vi "HIOKI PW3390 Conf Measure Item Harmonic.vi"(0 "VISA Resource":refnum<visa-resource-name>, 1 "LIST":T1={"LIST1"=[FALSE, FALSE, FALSE, FALSE, FALSE, FALSE, FALSE, FALSE], "LIST2"=[FALSE, FALSE, FALSE, FALSE, FALSE, FALSE, FALSE, FALSE], "LIST1 2"=[FALSE, FALSE, FALSE, FALSE, FALSE, FALSE, FALSE, FALSE], "LIST2 2"=[FALSE, FALSE, FALSE, FALSE, FALSE, FALSE, FALSE], "LIST1 3"=[FALSE, FALSE, FALSE, FALSE, FALSE, FALSE, FALSE, FALSE], "LIST2 3"=[FALSE, FALSE, FALSE, FALSE, FALSE, FALSE, FALSE]}, 2 "Min Order (0)":i32 min=0 max=100, 3 "Max Order (100)":i32=100 min=0 max=100, 4 "ODD/EVEN/ALL (2: ALL)":enum16{"ODD", "EVEN", "ALL"}(ring)=enum."ALL", 5 "error in (no error)":errorcluster, 6 "Set/Query (F: Set)":bool, 7 "OPC query (T: ON)":bool=TRUE, 8 "All Clear (F: Off)":bool, 9 "Error Out (F: Off)":bool) -> (14 "VISA Resource out":refnum<visa-resource-name>, 15 "LIST out":T1, 16 "Min Order out":i32, 17 "Max Order out":i32=100, 18 "ODD/EVEN/ALL out":enum16{"ODD", "EVEN", "ALL"}(ring)=enum."ALL", 19 "error out":errorcluster)   [LabVIEW 2009]
doc: "Set/Query\n Set: Send the setting commands for the device.\n Query: Query the setting of the device.\n\nAll Clear\n Initializes the harmonic communication output data items.\n All harmonic communication output data items become OFF.\n\nList\n Specify the Harmonic List (Level, Content, Phase Angle) .\n\nMin Order\n Sets the lower order value.\n Input Range: 0 - 100\nMax Order\n Sets the upper order value.\n Input Range: 0 - 100\n\nODD/EVEN/ALL\n Sets the harmonic order to output."
panel:
  # "Order"
  # "Order out"
  # "U1"
  # "U2"
  # "U3"
  # "U4"
  # "I1"
  # "I2"
  # "I3"
  # "I4"
  # "Level"
  # "P12"
  # "P123"
  # "P1"
  # "P2"
  # "P3"
  # "P4"
  # "P34"
  # "FREQ"
  # "U1"
  # "U2"
  # "U3"
  # "U4"
  # "I1"
  # "I2"
  # "I3"
  # "I4"
  # "%"
  # "P12"
  # "P123"
  # "P1"
  # "P2"
  # "P3"
  # "P4"
  # "P34"
  # "U1"
  # "U2"
  # "U3"
  # "U4"
  # "I1"
  # "I2"
  # "I3"
  # "I4"
  # "Phase"
  # "P12"
  # "P123"
  # "P1"
  # "P2"
  # "P3"
  # "P4"
  # "P34"
  # "U1"
  # "U2"
  # "U3"
  # "U4"
  # "I1"
  # "I2"
  # "I3"
  # "I4"
  # "Level"
  # "P12"
  # "P123"
  # "P1"
  # "P2"
  # "P3"
  # "P4"
  # "P34"
  # "FREQ"
  # "U1"
  # "U2"
  # "U3"
  # "U4"
  # "I1"
  # "I2"
  # "I3"
  # "I4"
  # "%"
  # "P12"
  # "P123"
  # "P1"
  # "P2"
  # "P3"
  # "P4"
  # "P34"
  # "U1"
  # "U2"
  # "U3"
  # "U4"
  # "I1"
  # "I2"
  # "I3"
  # "I4"
  # "Phase"
  # "P12"
  # "P123"
  # "P1"
  # "P2"
  # "P3"
  # "P4"
  # "P34"
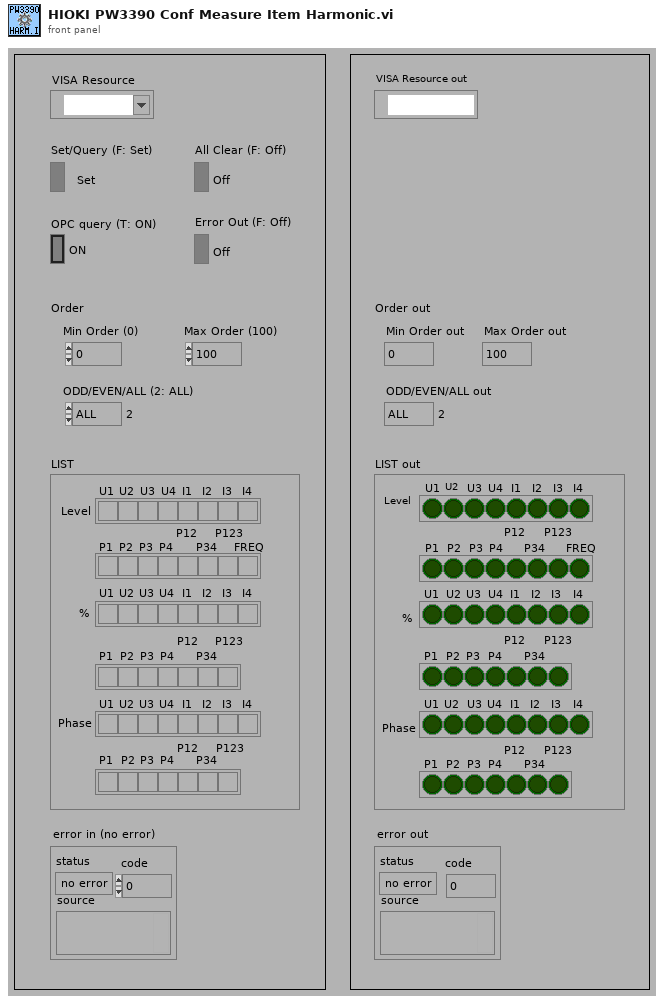
[diagram p1: front panel]
types:
  T1 = cluster{"LIST1":bool[], "LIST2":bool[], "LIST1 2":bool[], "LIST2 2":bool[], "LIST1 3":bool[], "LIST2 3":bool[]}
  T2 = cluster{"Boolean array":bool[], "Boolean array":bool[], "Boolean array":bool[], "Boolean array":bool[], "Boolean array":bool[], "Boolean array":bool[]}
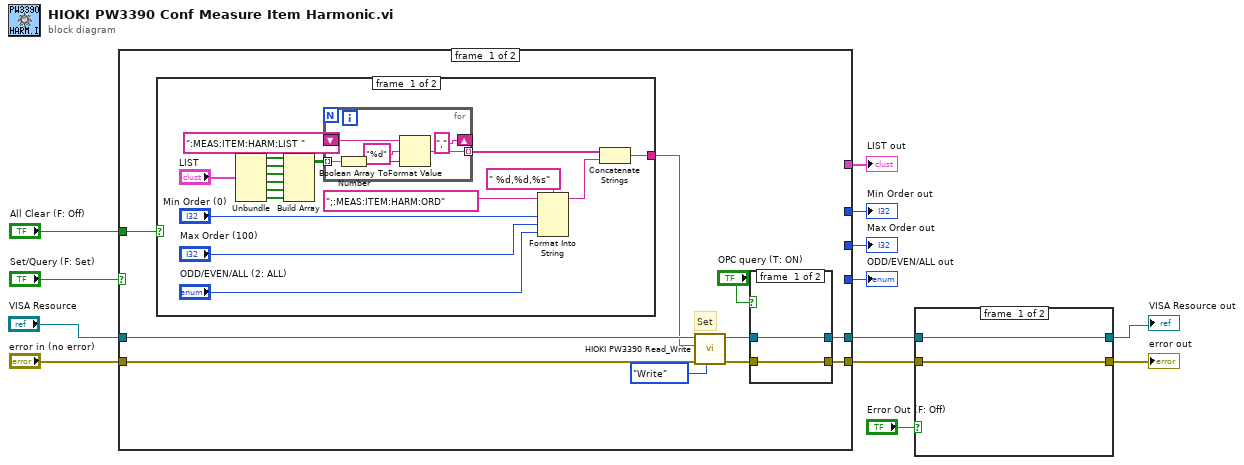
[diagram p0: block diagram]
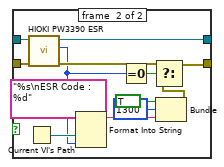
[diagram p2: hidden frame]
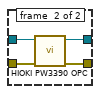
[diagram p3: hidden frame]
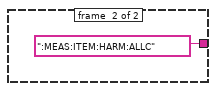
[diagram p4: hidden frame]
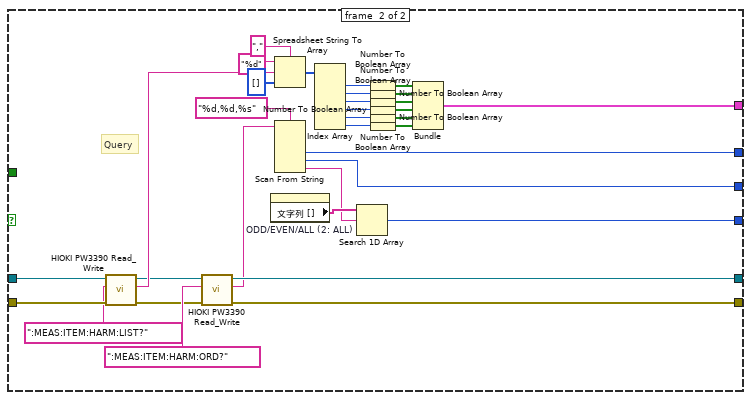
[diagram p5: hidden frame]
diagram:
  n1 = case shown="FALSE" "Set/Query (F: Set)" {
    tunnel: "error in (no error)" -> [w22 w85]
    tunnel: [w14 w78] -> w10
    tunnel: "VISA Resource" -> [w23 w86]
    tunnel: [w15 w75] -> w9
    tunnel: [_ w61] -> w7
    tunnel: [_ w56] -> w6
    tunnel: [_ w55] -> w5
    tunnel: [_ w54] -> w4
    tunnel: "All Clear (F: Off)" -> [w19 _]
    frame #0 {
      # "Set"
      n2 = case shown="FALSE" w19 {
        tunnel: [w30 ":MEAS:ITEM:HARM:ALLC"] -> w20
        frame #0 {
          n3 = Unbundle("LIST") -> ("LIST1"=w43:bool[], "LIST2"=w42:bool[], "LIST1 2"=w41:bool[], "LIST2 2"=w40:bool[], "LIST1 3"=w39:bool[], "LIST2 3"=w38:bool[])
          n4 = Build Array(w43, w42, w41, w40, w39, w38) -> (w46:bool[][])
          n5 = for {
            shift-right: [","] -> _
            shift-left: ":MEAS:ITEM:HARM:LIST " -> [w47]
            tunnel: [w48] -> w35 mode=indexing
            tunnel: w46 -> [w51] mode=indexing
            n6 = Boolean Array To Number(Boolean array=w51) -> (number=w50:u32)
            n7 = Format Value(string ("")=w47, format string="%d", value (0)=w50) -> (output string=w48:string)
          }
          n8 = Format Into String(format string=" %d,%d,%s", initial string=";:MEAS:ITEM:HARM:ORD", "Min Order (0)", "Max Order (100)", "ODD/EVEN/ALL (2: ALL)") -> (resulting string=w31:string)  [unwired: 1 in, 1 out]
          n9 = Concatenate Strings(w35, w31) -> (w30:string)
        }
        frame #1 {
        }
      }
      n10 = call <instrlib>:"HIOKI PW3390 Read_Write.vi"("Read/Write"=enum16{"Read", "Write"}."Write", "error in (no error)"=w22, "data in"=w20, "VISA Resource"=w23) -> ("error out"=w16:errorcluster, "VISA Resource out"=w17:refnum<visa-resource-name>)  [unwired: 5 in, 1 out]
      n11 = case shown="TRUE" "OPC query (T: ON)" {
        tunnel: [w25 w29] -> w15
        tunnel: [w24 w28] -> w14
        tunnel: w17 -> [w25 w27]
        tunnel: w16 -> [w24 w26]
        frame #0 {
        }
        frame #1 {
          n12 = call <instrlib>:"HIOKI PW3390 OPC.vi"("error in (no error)"=w26, "VISA Resource"=w27) -> ("error out"=w28:errorcluster, "VISA Resource out"=w29:refnum<visa-resource-name>)  [unwired: 7 in, 1 out]
        }
      }
    }
    frame #1 {
      # "Query"
      n13 = call <instrlib>:"HIOKI PW3390 Read_Write.vi"("error in (no error)"=w85, "data in"=":MEAS:ITEM:HARM:LIST?", "VISA Resource"=w86) -> ("error out"=w76:errorcluster, "data out"=w82:string, "VISA Resource out"=w77:refnum<visa-resource-name>)  [unwired: 6 in]
      n14 = call <instrlib>:"HIOKI PW3390 Read_Write.vi"("error in (no error)"=w76, "data in"=":MEAS:ITEM:HARM:ORD?", "VISA Resource"=w77) -> ("error out"=w78:errorcluster, "data out"=w57:string, "VISA Resource out"=w75:refnum<visa-resource-name>)  [unwired: 6 in]
      n15 = property on="ODD/EVEN/ALL (2: ALL)" class="Enum (strict)"() -> ("文字列 []"=w59:string[])  [unwired: 2 in, 2 out]
      n16 = Spreadsheet String To Array(delimiter (Tab)="," ("デリミタ（Tab）"), format string="%d" ("形式文字列"), spreadsheet string=w82, array type (2D Dbl)=u8[] []) -> (array=w74:u8[])
      n17 = Scan From String(format string="%d,%d,%s" ("形式文字列"), input string=w57) -> (output 1=w56:i32, output 2=w55:i32, output 3=w58:string)  [unwired: 5 in, 3 out]
      n18 = Index Array(array=w74) -> (element #1=w73:u8, element #2=w72:u8, element #3=w71:u8, element #4=w70:u8, element #5=w69:u8, element #6=w68:u8)  [unwired: 6 in]
      n19 = Search 1D Array(1D array=w59, element=w58) -> (index of element=w54:i32)  [unwired: 1 in]
      n20 = Number To Boolean Array(number=w73) -> (Boolean array=w67:bool[])
      n21 = Number To Boolean Array(number=w72) -> (Boolean array=w66:bool[])
      n22 = Number To Boolean Array(number=w71) -> (Boolean array=w65:bool[])
      n23 = Number To Boolean Array(number=w70) -> (Boolean array=w64:bool[])
      n24 = Number To Boolean Array(number=w69) -> (Boolean array=w63:bool[])
      n25 = Number To Boolean Array(number=w68) -> (Boolean array=w62:bool[])
      n26 = Bundle("Boolean array"=w67, "Boolean array"=w66, "Boolean array"=w65, "Boolean array"=w64, "Boolean array"=w63, "Boolean array"=w62) -> (w61:T2)  [unwired: 1 in]
    }
  }
  "Max Order out" <- w5
  "Min Order out" <- w6
  "LIST out" <- w7
  "ODD/EVEN/ALL out" <- w4
  n27 = case shown="TRUE" "Error Out (F: Off)" {
    tunnel: w9 -> [w88 w101]
    tunnel: w10 -> [w87 w100]
    tunnel: [w87 w90] -> w8
    tunnel: [w88 w99] -> w1
    frame #0 {
    }
    frame #1 {
      n28 = Current VI's Path() -> (path=w97:path)
      n29 = call <instrlib>:"HIOKI PW3390 ESR.vi"("error in (no error)"=w100, "VISA Resource"=w101) -> ("error out"=w91:errorcluster, "Output Value"=w89:u8, "VISA Resource out"=w99:refnum<visa-resource-name>)  [unwired: 6 in, 1 out]
      n30 = Format Into String(format string="%s\nESR Code : %d", w97, w89) -> (resulting string=w93:string)  [unwired: 2 in, 1 out]
      n31 = Equal To 0?(x=w89) -> (x = 0?=w98:bool)
      n32 = Bundle("status"=TRUE, "code"=1300, w93) -> (w92:cluster{"status":bool, "code":i32, string})  [unwired: 1 in]
      n33 = Select(t=w91, s=w98, f=w92) -> (s? t:f=w90:errorcluster)
    }
  }
  "error out" <- w8
  "VISA Resource out" <- w1
